vi "getLaserPower.vi"(8 "error in (no error)":errorcluster, 11 "Monochromator in":refnum<class "Monochromator.lvclass">) -> (0 "error out":errorcluster, 2 "power":dbl, 3 "Monochromator out":refnum<class "Monochromator.lvclass">)   [LabVIEW 2023, in "Monochromator.lvclass"]
uses:
  Monochromator.lvclass
  d9b87029-586e-44ee-a6e5-d4a5e0edce38.vi
  b59fd1e7-dcda-425c-bd6c-61aafb79e7f4.vi
  <vilib>/JDP Science/JSONtext/Variant to JSON Text.vi
  <vilib>/JDP Science/JSONtext/Set Item.vi
  <vilib>/JDP Science/JSONtext/JSON text to Variant.vi
  <vilib>/JDP Science/JSONtext/LVClass Serializer/JSONtext LVClass Serializer.lvclass
  Monochromator.lvclass/Monochromator.ctl
  GenericDevice/GenericDevice.lvclass
  <vilib>/IlluminatedG/lv-web-crypto/lv-json/JSON/JSON.lvlib
  LaserPower.ctl
panel:
  # "Connector Pane"
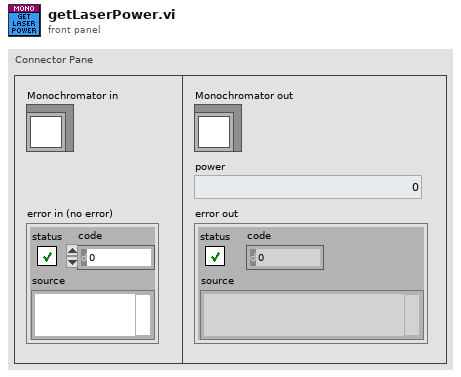
[diagram p1: front panel]
types:
  T1 = typedef "Monochromator.lvclass/LaserPower.ctl" = cluster{"power":dbl}
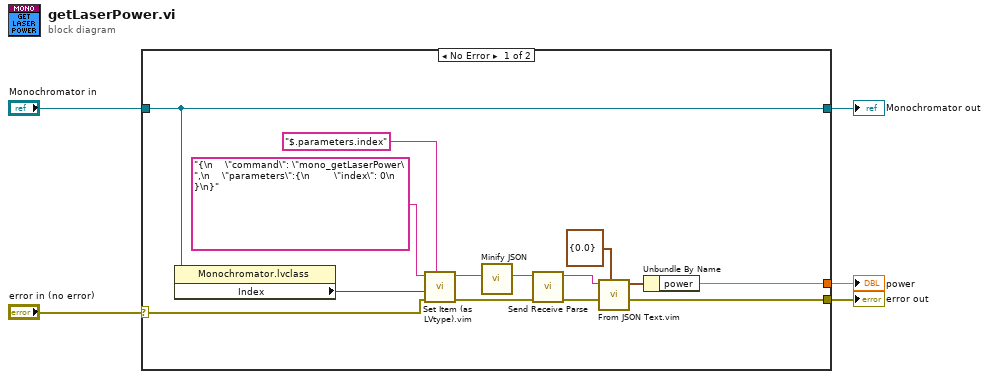
[diagram p0: block diagram]
diagram:
  n1 = case shown="No Error" "error in (no error)" {
    selector: "error in (no error)" -> [w15 w21]
    tunnel: [w14 w21] -> w4
    tunnel: [w17 w20] -> w2
    tunnel: "Monochromator in" -> [w17 w20]
    tunnel: [w6 _] -> w1
    frame No Error {
      n2 = property class="Monochromator.lvclass"(reference=w17) -> ("Index"=w16:i32)  [unwired: 1 in, 2 out]
      n3 = call "Set Item (as LVtype).vim"("$Path or Item Name"="$.parameters.index", "error in (no error)"=w15, "Anything"=w16, "JSON"="{\n    \"command\": \"mono_getLaserPower\",\n    \"parameters\":{\n        \"index\": 0\n    }\n}") -> ("error out"=w13:errorcluster, "<JSON>"=w10:string)  [unwired: 4 in, 1 out]
      n4 = call <vilib>:"Minify JSON.vi"("JSON String"=w10) -> ("Minified JSON"=w9:string)  [unwired: 10 in]
      n5 = call "Send Receive Parse.vi"("error in"=w13, "<JSON>"=w9) -> ("error out"=w11:errorcluster, "results-JSON string"=w12:string)  [unwired: 7 in, 1 out]
      n6 = call "From JSON Text.vim"("Data Type and Default Value"=T1 {"power"=0.0} ("Laser Power"), "error in (no error)"=w11, "JSON"=w12) -> ("error out"=w14:errorcluster, "Data out"=w7:T1)  [unwired: 7 in]
      n7 = Unbundle By Name(w7) -> ("power"=w6:dbl)
    }
    frame Error {
    }
  }
  "error out" <- w4
  "Monochromator out" <- w2
  "power" <- w1
